vi "Error_Helper_BuildCluster.vi"(6 "Additional Info":string, 8 "Error In":errorcluster, 11 "Code":i32) -> (0 "Error Out":errorcluster)   [LabVIEW 2022 SP3, in "hse-misc.lvlib"]
doc: "Builds an error cluster from <b>Code</b> and <b>Additional Info</b>\n\n____\nHAMPEL SOFTWARE ENGINEERING v3.8.0 (2023-12-18 14:41)"
uses:
  hse-misc.lvlib
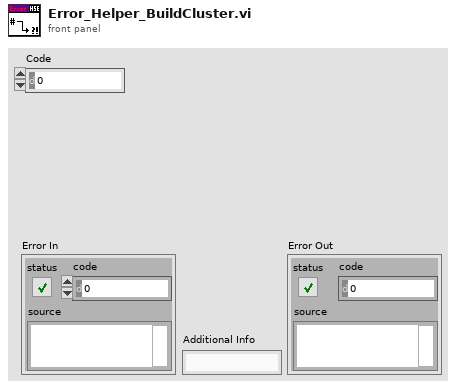
[diagram p1: front panel]
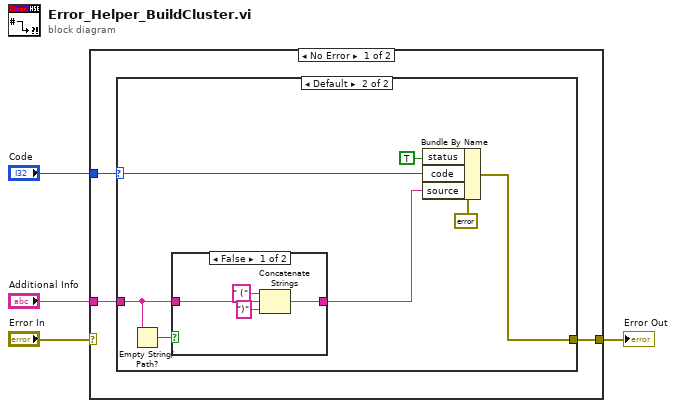
[diagram p0: block diagram]
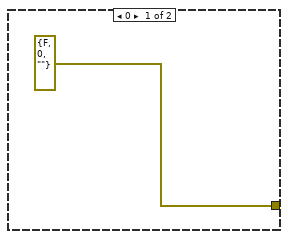
[diagram p2: hidden frame]
diagram:
  n1 = case shown="No Error" "Error In" {
    selector: "Error In" -> [_ w21]
    tunnel: [w7 w21] -> w4
    tunnel: "Code" -> [w6 _]
    tunnel: "Additional Info" -> [w5 _]
    frame No Error {
      n2 = case shown="Default" w6 {
        selector: w6 -> [_ w12]
        tunnel: [errorcluster {"status"=FALSE, "code"=0, "source"=""} ("error IO") w15] -> w7
        tunnel: w5 -> [_ w10]
        frame 0 {
        }
        frame Default {
          n3 = Empty String/Path?(string/path=w10) -> (empty?=w11:bool)
          n4 = case shown="False" w11 {
            tunnel: w10 -> [w19 w20]
            tunnel: [w18 w20] -> w9
            frame False {
              n5 = Concatenate Strings(" (" ("string"), w19, ")" ("string")) -> (w18:string)
            }
            frame True {
            }
          }
          n6 = Bundle By Name(cluster=errorcluster {"status"=TRUE, "code"=0, "source"=""} ("error IO"), "status"=TRUE, "code"=w12, "source"=w9) -> (w15:errorcluster)
        }
      }
    }
    frame Error {
    }
  }
  "Error Out" <- w4
